vi "AC Get Image v2.vi"() -> (3 "AC Image":sgl[][](array[numeric]))   [LabVIEW 2014]
panel:
  out "Current Image":sgl[][](graph)
  in  "Save Data":bool
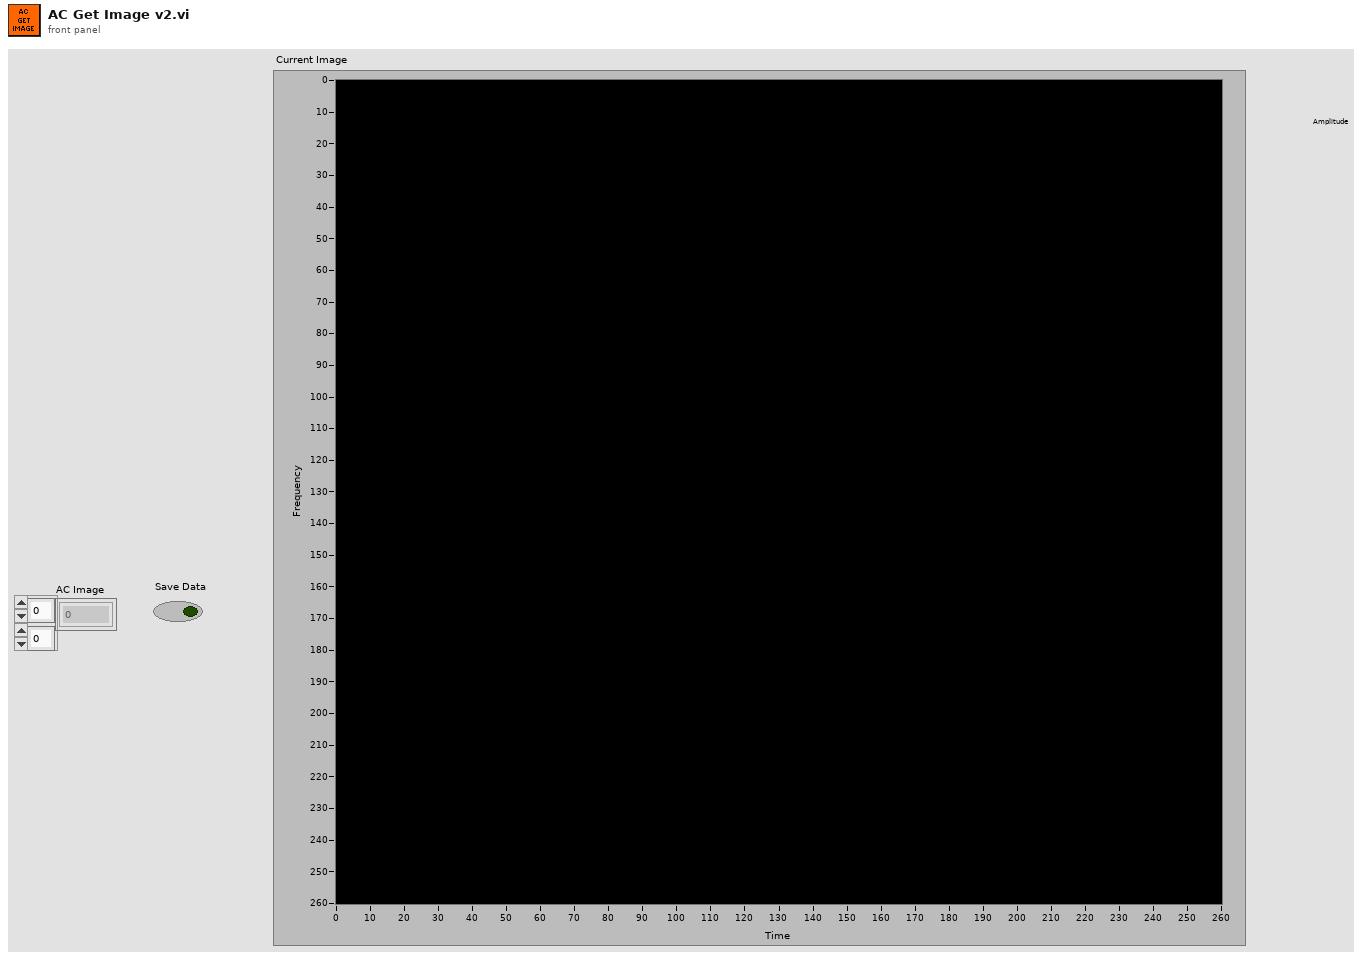
[diagram p1: front panel]
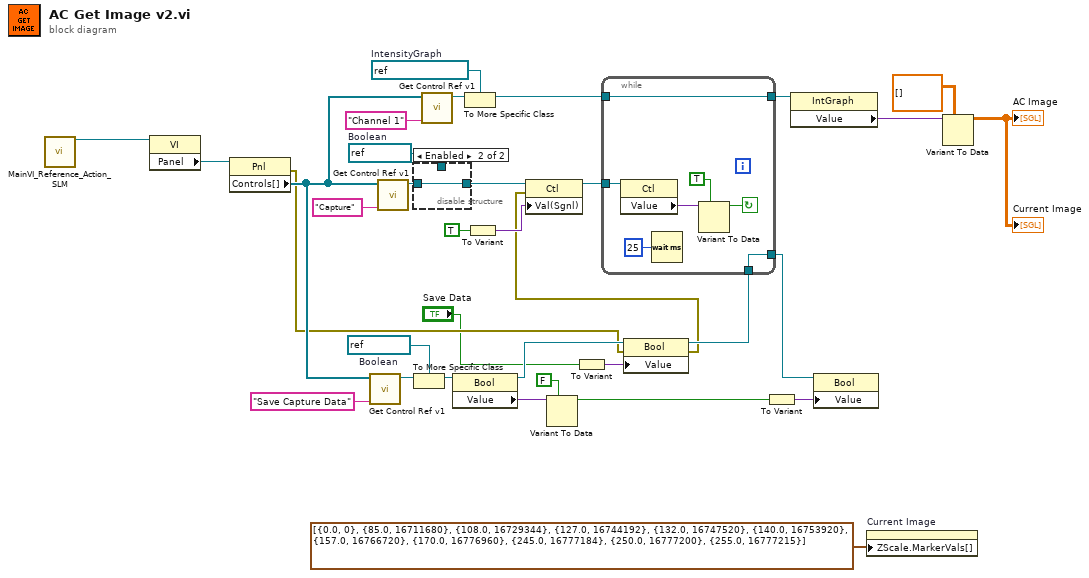
[diagram p0: block diagram]
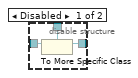
[diagram p2: hidden frame]
diagram:
  w16 = refnum<vi> refnum  # Boolean
  w24 = refnum<vi> refnum  # IntensityGraph
  w30 = refnum<vi> refnum  # Boolean
  n1 = call "MainVI_Reference_Action_SLM.vi"() -> ("VI Reference"=w34:refnum<vi>)  [unwired: 15 in]
  n2 = property class="VI"(reference=w34) -> ("Panel"=w33:refnum<vi>)  [unwired: 1 in, 2 out]
  n3 = property class="Pnl"(reference=w33) -> (error out=w5:errorcluster, "Controls[]"=w17:refnum<vi>[])  [unwired: 1 in, 1 out]
  n4 = call "Get Control Ref v1.vi"("Control Name"="Save Capture Data", "Controls Array"=w17) -> ("Ctl Refnum Out"=w15:refnum<vi>)  [unwired: 9 in]
  n5 = call "Get Control Ref v1.vi"("Control Name"="Capture", "Controls Array"=w17) -> ("Ctl Refnum Out"=w31:refnum<vi>)  [unwired: 9 in]
  n6 = disable-structure shown="Enabled" {
    disable-tunnel: w31 -> [w37 w38]
    disable-tunnel: w30 -> [w36 _]
    disable-tunnel: [w35 w38] -> w29
    frame Disabled {
      n7 = To More Specific Class(target class=w36, reference=w37) -> (specific class reference=w35:refnum<vi>)  [unwired: 1 in, 1 out]
    }
    frame Enabled {
    }
  }
  n8 = To More Specific Class(target class=w16, reference=w15) -> (specific class reference=w14:refnum<vi>)  [unwired: 1 in, 1 out]
  n9 = call "Get Control Ref v1.vi"("Control Name"="Channel 1", "Controls Array"=w17) -> ("Ctl Refnum Out"=w23:refnum<vi>)  [unwired: 9 in]
  n10 = property class="Bool"(reference=w14) -> (reference out=w12:refnum<vi>, "Value"=w13:variant)  [unwired: 1 in, 1 out]
  n11 = To More Specific Class(target class=w24, reference=w23) -> (specific class reference=w22:refnum<vi>)  [unwired: 1 in, 1 out]
  n12 = To Variant(anything=TRUE) -> (Variant=w27:variant)
  n13 = Variant To Data(type=FALSE, Variant=w13) -> (data=w6:bool)  [unwired: 1 in, 1 out]
  n14 = To Variant(anything="Save Data") -> (Variant=w11:variant)
  n15 = property class="Bool"(reference=w12, error in=w5, "Value"=w11) -> (reference out=w9:refnum<vi>, error out=w4:errorcluster)
  n16 = property class="Ctl"(reference=w29, error in=w4, "Val(Sgnl)"=w27) -> (reference out=w26:refnum<vi>)  [unwired: 1 out]
  n17 = while {
    tunnel: w26 -> [w45]
    tunnel: w22 -> [w40]
    tunnel: [w40] -> w21
    tunnel: w9 -> [w39]
    tunnel: [w39] -> w7
    stop <- w42 continue-if-true
    n18 = property class="Ctl"(reference=w45) -> ("Value"=w44:variant)  [unwired: 1 in, 2 out]
    n19 = Wait (ms)(milliseconds to wait=u32 25) -> ()  [unwired: 1 out]
    n20 = Variant To Data(type=TRUE, Variant=w44) -> (data=w42:bool)  [unwired: 1 in, 1 out]
  }
  n21 = To Variant(anything=w6) -> (Variant=w8:variant)
  n22 = property class="IntGraph"(reference=w21) -> ("Value"=w20:variant)  [unwired: 1 in, 2 out]
  n23 = property class="Bool"(reference=w7, "Value"=w8) -> ()  [unwired: 1 in, 2 out]
  n24 = property on="Current Image" class="IntGraph (strict)"("ZScale.MarkerVals[]"=cluster{dbl, u32}[] [{0.0, 0}, {85.0, 16711680}, {108.0, 16729344}, {127.0, 16744192}, {132.0, 16747520}, {140.0, 16753920}, {157.0, 16766720}, {170.0, 16776960}, {245.0, 16777184}, {250.0, 16777200}, {255.0, 16777215}] ("Z Scale.Marker Values[]")) -> ()  [unwired: 2 in, 2 out]
  n25 = Variant To Data(type=sgl[][] [], Variant=w20) -> (data=→"AC Image" →"Current Image":sgl[][])  [unwired: 1 in, 1 out]
